vi "Modify VI Window Dimensions.vi"(9 "time (ms)":i32=250, 10 "x":u32, 11 "Action on x":T1(ring)) -> ()   [LabVIEW 2011]
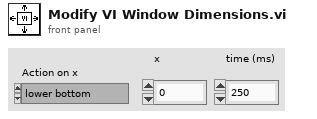
[diagram p1: front panel]
types:
  T1 = enum16{"lower bottom", "raise bottom", "lower top", "raise top", "extend right", "reduce right", "extend left", "reduce left"}
  T2 = typedef "LVRectTypeDef.ctl" = cluster{"left":i16, "top":i16, "right":i16, "bottom":i16}
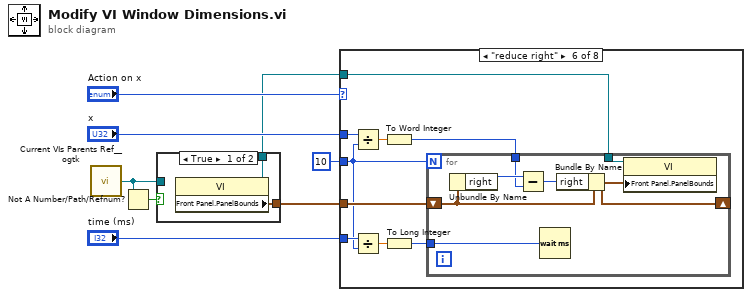
[diagram p0: block diagram]
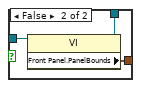
[diagram p2: hidden frame]
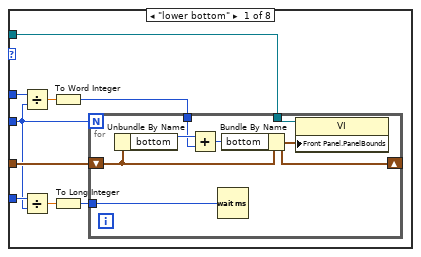
[diagram p3: hidden frame]
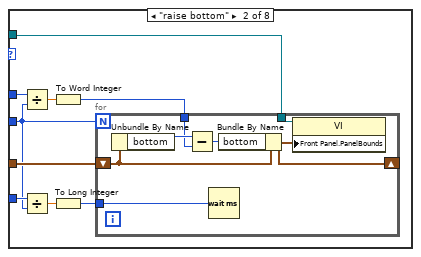
[diagram p4: hidden frame]
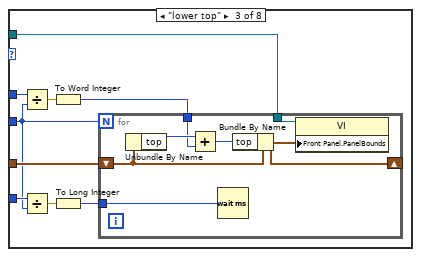
[diagram p5: hidden frame]
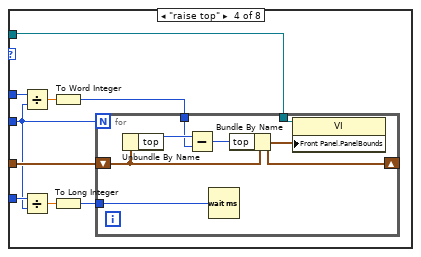
[diagram p6: hidden frame]
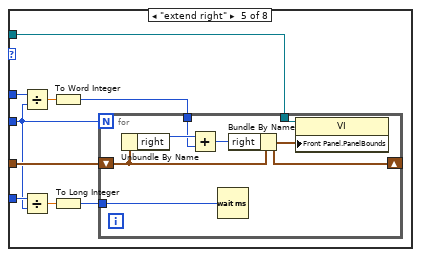
[diagram p7: hidden frame]
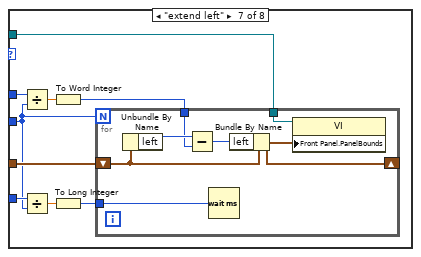
[diagram p8: hidden frame]
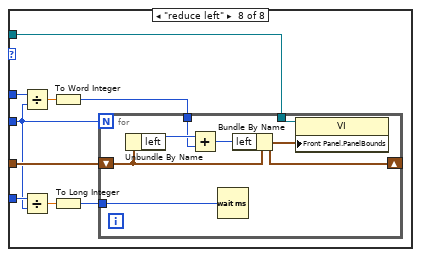
[diagram p9: hidden frame]
diagram:
  n1 = call "Current VIs Parents Ref__ogtk.vi"() -> ("Calling VI's Reference"=w1:refnum<vi>)  [unwired: 2 in]
  n2 = Not A Number/Path/Refnum?(number/path/refnum=w1) -> (NaN/Path/Refnum?=w2:bool)
  n3 = case shown="True" w2 {
    tunnel: [w10 w13] -> w8
    tunnel: w1 -> [_ w12]
    tunnel: [w9 w11] -> w3
    frame True {
      n4 = property class="VI"() -> (reference out=w9:refnum<vi>, "Front Panel.PanelBounds"=w10:T2)  [unwired: 2 in, 1 out]
    }
    frame False {
      n5 = property class="VI"(reference=w12) -> (reference out=w11:refnum<vi>, "Front Panel.PanelBounds"=w13:T2)  [unwired: 1 in, 1 out]
    }
  }
  n6 = case shown="\"reduce right\"" "Action on x" {
    tunnel: w8 -> [w22 w38 w54 w70 w86 w102 w118 w134]
    tunnel: "x" -> [w19 w35 w51 w67 w83 w99 w115 w131]
    tunnel: "time (ms)" -> [w17 w34 w49 w66 w81 w98 w114 w129]
    tunnel: 10 ("iterations") -> [w16 w33 w48 w65 w80 w97 w113 w128]
    tunnel: w3 -> [w14 w30 w46 w62 w78 w94 w110 w126]
    frame "lower bottom" {
      n7 = Divide(x=w19, y=w16) -> (x/y=w21:dbl)
      n8 = Divide(x=w17, y=w16) -> (x/y=w20:dbl)
      n9 = To Word Integer(number=w21) -> (16bit integer=w18:i16)
      n10 = To Long Integer(number=w20) -> (32bit integer=w15:i32)
      n11 = for {
        N: w16 -> [_]
        shift-right: [w26] -> _
        shift-left: w22 -> [w28]
        tunnel: w18 -> [w25]
        tunnel: w15 -> [w24]
        tunnel: w14 -> [w23]
        n12 = Unbundle By Name(w28) -> ("bottom"=w27:i16)
        n13 = Add(x=w27, y=w25) -> (x+y=w29:i16)
        n14 = Wait (ms)(milliseconds to wait=w24) -> ()  [unwired: 1 out]
        n15 = Bundle By Name(cluster=w28, "bottom"=w29) -> (w26:T2)
        n16 = property class="VI"(reference=w23, "Front Panel.PanelBounds"=w26) -> ()  [unwired: 1 in, 2 out]
      }
    }
    frame "raise bottom" {
      n17 = Divide(x=w35, y=w33) -> (x/y=w37:dbl)
      n18 = Divide(x=w34, y=w33) -> (x/y=w32:dbl)
      n19 = To Word Integer(number=w37) -> (16bit integer=w36:i16)
      n20 = To Long Integer(number=w32) -> (32bit integer=w31:i32)
      n21 = for {
        N: w33 -> [_]
        shift-right: [w42] -> _
        shift-left: w38 -> [w44]
        tunnel: w36 -> [w41]
        tunnel: w31 -> [w40]
        tunnel: w30 -> [w39]
        n22 = Unbundle By Name(w44) -> ("bottom"=w43:i16)
        n23 = Subtract(x=w43, y=w41) -> (x-y=w45:i16)
        n24 = Wait (ms)(milliseconds to wait=w40) -> ()  [unwired: 1 out]
        n25 = Bundle By Name(cluster=w44, "bottom"=w45) -> (w42:T2)
        n26 = property class="VI"(reference=w39, "Front Panel.PanelBounds"=w42) -> ()  [unwired: 1 in, 2 out]
      }
    }
    frame "lower top" {
      n27 = Divide(x=w51, y=w48) -> (x/y=w53:dbl)
      n28 = Divide(x=w49, y=w48) -> (x/y=w52:dbl)
      n29 = To Word Integer(number=w53) -> (16bit integer=w50:i16)
      n30 = To Long Integer(number=w52) -> (32bit integer=w47:i32)
      n31 = for {
        N: w48 -> [_]
        shift-right: [w58] -> _
        shift-left: w54 -> [w60]
        tunnel: w50 -> [w57]
        tunnel: w47 -> [w56]
        tunnel: w46 -> [w55]
        n32 = Unbundle By Name(w60) -> ("top"=w59:i16)
        n33 = Add(x=w59, y=w57) -> (x+y=w61:i16)
        n34 = Wait (ms)(milliseconds to wait=w56) -> ()  [unwired: 1 out]
        n35 = Bundle By Name(cluster=w60, "top"=w61) -> (w58:T2)
        n36 = property class="VI"(reference=w55, "Front Panel.PanelBounds"=w58) -> ()  [unwired: 1 in, 2 out]
      }
    }
    frame "raise top" {
      n37 = Divide(x=w67, y=w65) -> (x/y=w69:dbl)
      n38 = Divide(x=w66, y=w65) -> (x/y=w64:dbl)
      n39 = To Word Integer(number=w69) -> (16bit integer=w68:i16)
      n40 = To Long Integer(number=w64) -> (32bit integer=w63:i32)
      n41 = for {
        N: w65 -> [_]
        shift-right: [w74] -> _
        shift-left: w70 -> [w76]
        tunnel: w68 -> [w73]
        tunnel: w63 -> [w72]
        tunnel: w62 -> [w71]
        n42 = Unbundle By Name(w76) -> ("top"=w75:i16)
        n43 = Subtract(x=w75, y=w73) -> (x-y=w77:i16)
        n44 = Wait (ms)(milliseconds to wait=w72) -> ()  [unwired: 1 out]
        n45 = Bundle By Name(cluster=w76, "top"=w77) -> (w74:T2)
        n46 = property class="VI"(reference=w71, "Front Panel.PanelBounds"=w74) -> ()  [unwired: 1 in, 2 out]
      }
    }
    frame "extend right" {
      n47 = Divide(x=w83, y=w80) -> (x/y=w85:dbl)
      n48 = Divide(x=w81, y=w80) -> (x/y=w84:dbl)
      n49 = To Word Integer(number=w85) -> (16bit integer=w82:i16)
      n50 = To Long Integer(number=w84) -> (32bit integer=w79:i32)
      n51 = for {
        N: w80 -> [_]
        shift-right: [w90] -> _
        shift-left: w86 -> [w92]
        tunnel: w82 -> [w89]
        tunnel: w79 -> [w88]
        tunnel: w78 -> [w87]
        n52 = Unbundle By Name(w92) -> ("right"=w91:i16)
        n53 = Add(x=w91, y=w89) -> (x+y=w93:i16)
        n54 = Wait (ms)(milliseconds to wait=w88) -> ()  [unwired: 1 out]
        n55 = Bundle By Name(cluster=w92, "right"=w93) -> (w90:T2)
        n56 = property class="VI"(reference=w87, "Front Panel.PanelBounds"=w90) -> ()  [unwired: 1 in, 2 out]
      }
    }
    frame "reduce right" {
      n57 = Divide(x=w99, y=w97) -> (x/y=w101:dbl)
      n58 = Divide(x=w98, y=w97) -> (x/y=w96:dbl)
      n59 = To Word Integer(number=w101) -> (16bit integer=w100:i16)
      n60 = To Long Integer(number=w96) -> (32bit integer=w95:i32)
      n61 = for {
        N: w97 -> [_]
        shift-right: [w106] -> _
        shift-left: w102 -> [w108]
        tunnel: w100 -> [w105]
        tunnel: w95 -> [w104]
        tunnel: w94 -> [w103]
        n62 = Unbundle By Name(w108) -> ("right"=w107:i16)
        n63 = Subtract(x=w107, y=w105) -> (x-y=w109:i16)
        n64 = Wait (ms)(milliseconds to wait=w104) -> ()  [unwired: 1 out]
        n65 = Bundle By Name(cluster=w108, "right"=w109) -> (w106:T2)
        n66 = property class="VI"(reference=w103, "Front Panel.PanelBounds"=w106) -> ()  [unwired: 1 in, 2 out]
      }
    }
    frame "extend left" {
      n67 = Divide(x=w115, y=w113) -> (x/y=w117:dbl)
      n68 = Divide(x=w114, y=w113) -> (x/y=w112:dbl)
      n69 = To Word Integer(number=w117) -> (16bit integer=w116:i16)
      n70 = To Long Integer(number=w112) -> (32bit integer=w111:i32)
      n71 = for {
        N: w113 -> [_]
        shift-right: [w122] -> _
        shift-left: w118 -> [w124]
        tunnel: w116 -> [w121]
        tunnel: w111 -> [w120]
        tunnel: w110 -> [w119]
        n72 = Unbundle By Name(w124) -> ("left"=w123:i16)
        n73 = Subtract(x=w123, y=w121) -> (x-y=w125:i16)
        n74 = Wait (ms)(milliseconds to wait=w120) -> ()  [unwired: 1 out]
        n75 = Bundle By Name(cluster=w124, "left"=w125) -> (w122:T2)
        n76 = property class="VI"(reference=w119, "Front Panel.PanelBounds"=w122) -> ()  [unwired: 1 in, 2 out]
      }
    }
    frame "reduce left" {
      n77 = Divide(x=w131, y=w128) -> (x/y=w133:dbl)
      n78 = Divide(x=w129, y=w128) -> (x/y=w132:dbl)
      n79 = To Word Integer(number=w133) -> (16bit integer=w130:i16)
      n80 = To Long Integer(number=w132) -> (32bit integer=w127:i32)
      n81 = for {
        N: w128 -> [_]
        shift-right: [w138] -> _
        shift-left: w134 -> [w140]
        tunnel: w130 -> [w137]
        tunnel: w127 -> [w136]
        tunnel: w126 -> [w135]
        n82 = Unbundle By Name(w140) -> ("left"=w139:i16)
        n83 = Add(x=w139, y=w137) -> (x+y=w141:i16)
        n84 = Wait (ms)(milliseconds to wait=w136) -> ()  [unwired: 1 out]
        n85 = Bundle By Name(cluster=w140, "left"=w141) -> (w138:T2)
        n86 = property class="VI"(reference=w135, "Front Panel.PanelBounds"=w138) -> ()  [unwired: 1 in, 2 out]
      }
    }
  }
